vi "ArmMath(SubVI).vi"(9 "Hight(Inches)":dbl, 10 "Arm length":dbl, 11 "Arm Hight":dbl) -> (3 "Angle":dbl)   [LabVIEW 2018, in "Elevator.lvlib" / "Elevator.lvclass"]
uses:
  Elevator.lvclass
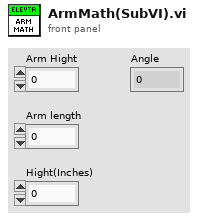
[diagram p1: front panel]
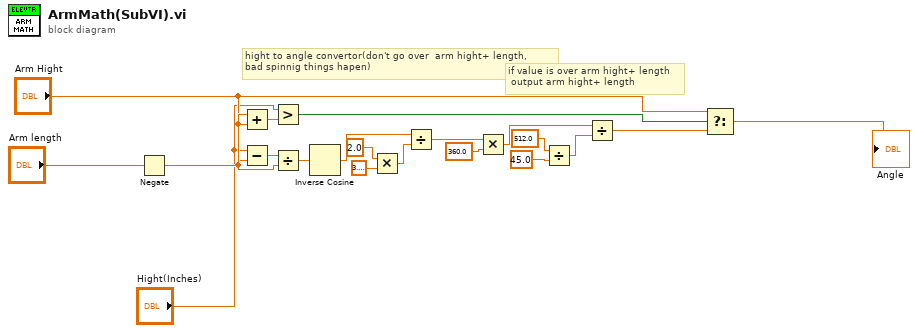
[diagram p0: block diagram]
diagram:
  # "if value is over arm hight+ length\n output arm hight+ length"
  # "hight to angle convertor(don't go over  arm hight+ length, \nbad spinnig things hapen)"
  n1 = Negate(x="Arm length") -> (-x=w20:dbl)
  n2 = Add(x=w20, y="Arm Hight") -> (x+y=w6:dbl)
  n3 = Subtract(x="Hight(Inches)", y="Arm Hight") -> (x-y=w1:dbl)
  n4 = Greater?(x="Hight(Inches)", y=w6) -> (0:w9:bool)
  n5 = Divide(x=w1, y=w20) -> (x/y=w2:dbl)
  n6 = Inverse Cosine(1:w2) -> (0:w17:dbl)
  n7 = Multiply(x=2.0, y=3.141592653589793) -> (x*y=w12:dbl)
  n8 = Divide(x=w17, y=w12) -> (x/y=w15:dbl)
  n9 = Multiply(x=w15, y=360.0) -> (x*y=w18:dbl)
  n10 = Divide(x=512.0, y=45.0) -> (x/y=w3:dbl)
  n11 = Divide(x=w18, y=w3) -> (x/y=w10:dbl)
  n12 = Select(t="Arm Hight", s=w9, f=w10) -> (s? t:f=→"Angle":dbl)
